vi "Init and Rotate array Graf3.vi"(5 "Reset":bool, 7 "Stop read":bool, 9 "Array size":i32=30, 10 "PV":dbl[](array[numeric]), 11 "XY Graf in":cluster{"time stamp":timestamp[], "PV":dbl[]}[](array[cluster])) -> (3 "XY Graf out":cluster{"time stamp":timestamp[], "PV":dbl[]}[](array[cluster]))   [LabVIEW 2019]
panel:
  out "XY Graf out 2":cluster{"time stamp":timestamp[], "PV":dbl[]}[](array[cluster])
  in  "XY Graf in 2":cluster{"time stamp":timestamp[], "PV":dbl[]}[](array[cluster])
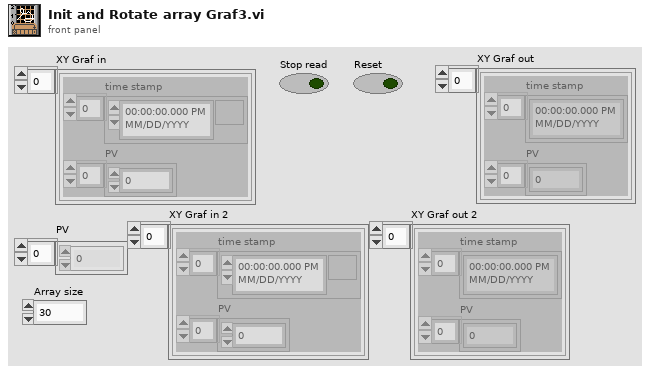
[diagram p1: front panel]
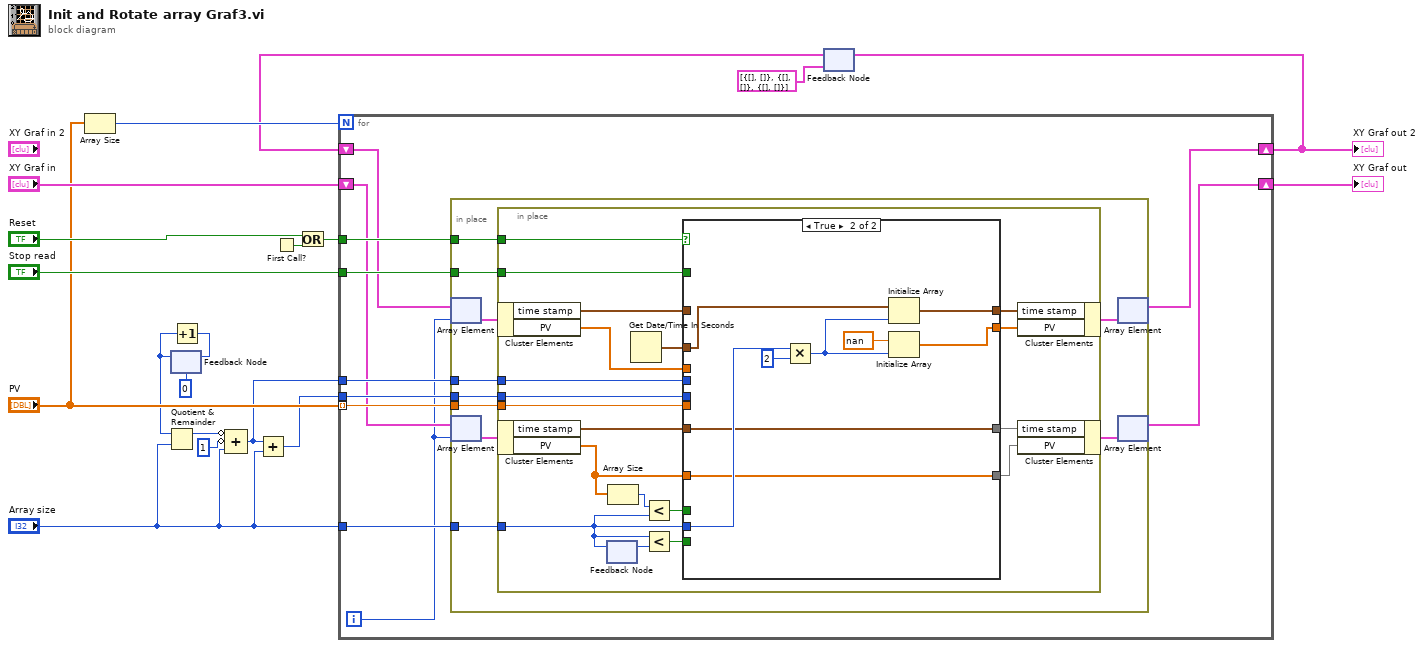
[diagram p0: block diagram]
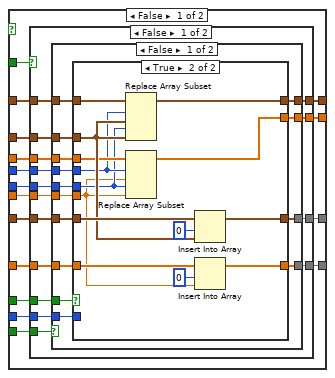
[diagram p2: hidden frame]
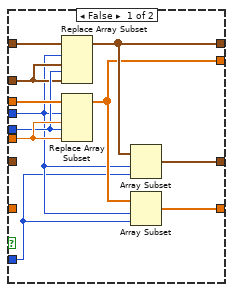
[diagram p3: hidden frame]
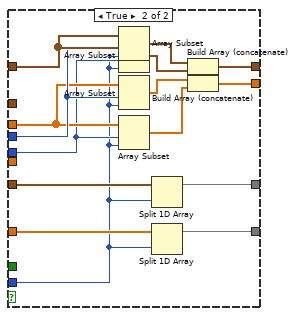
[diagram p4: hidden frame]
diagram:
  n1 = Array Size(array="PV") -> (size(s)=w15:i32)
  n2 = feedback #1(0 ("t")) -> (w11:i32)
  n3 = Quotient & Remainder(x=w11, y="Array size") -> (x-y*floor(x/y)=w10:i32)  [unwired: 1 out]
  n4 = Increment(x=w11) -> (x+1=w12:i32)
  n5 = feedback-in #1(w12) -> ()
  n6 = Compound Arithmetic op=ADD(invert w10, invert 1 ("value"), "Array size") -> (w7:i32)
  n7 = Add(x=w7, y="Array size") -> (x+y=w6:i32)
  n8 = First Call?() -> (First Call?: T/F=w4:bool)
  n9 = Or(x="Reset", y=w4) -> (x .or. y?=w5:bool)
  n10 = feedback #2(cluster{"time stamp":timestamp[], "PV":dbl[]}[] [{"time stamp"=[], "PV"=[]}, {"time stamp"=[], "PV"=[]}, {"time stamp"=[], "PV"=[]}] ("XY Graf out")) -> (w2:cluster{"time stamp":timestamp[], "PV":dbl[]}[])
  n11 = for {
    N: w15 -> [_]
    tunnel: "Stop read" -> [w30]
    tunnel: w5 -> [w29]
    tunnel: "PV" -> [w28] mode=indexing
    tunnel: "Array size" -> [w27]
    shift-right: [w20] -> w17
    shift-left: "XY Graf in" -> [w24]
    shift-right: [w21] -> w3
    shift-left: w2 -> [w23]
    tunnel: w7 -> [w26]
    tunnel: w6 -> [w25]
    i -> [w22]
    n12 = in-place {
      in-place-border: w30 -> [w40]
      in-place-border: w29 -> [w39]
      in-place-border: w28 -> [w38]
      in-place-border: w27 -> [w37]
      in-place-border: w26 -> [w36]
      in-place-border: w25 -> [w35]
      n13 = in-place-array #3(w23, w22) -> (w32:cluster{"time stamp":timestamp[], "PV":dbl[]})
      n14 = in-place-array #4(w24, w22) -> (w33:cluster{"time stamp":timestamp[], "PV":dbl[]})
      n15 = in-place {
        in-place-border: w40 -> [w59]
        in-place-border: w39 -> [w54]
        in-place-border: w38 -> [w57]
        in-place-border: w37 -> [w50]
        in-place-border: w36 -> [w44]
        in-place-border: w35 -> [w43]
        n16 = in-place-cluster #5(w32) -> ("time stamp"=w46:timestamp[], "PV"=w42:dbl[])
        n17 = in-place-cluster #6(w33) -> ("time stamp"=w55:timestamp[], "PV"=w49:dbl[])
        n18 = feedback #7() -> (w53:i32)  [unwired: 1 in]
        n19 = feedback-in #7(w50) -> ()
        n20 = Array Size(array=w49) -> (size(s)=w58:i32)
        n21 = Get Date/Time In Seconds() -> (seconds since 1Jan1904=w56:timestamp)
        n22 = Less?(x=w58, y=w50) -> (x < y?=w48:bool)
        n23 = Less?(x=w50, y=w53) -> (x < y?=w52:bool)
        n24 = case shown="True" w54 {
          tunnel: w59 -> [w67 _]
          tunnel: w57 -> [w75 _]
          tunnel: w56 -> [w74 w157]
          tunnel: [w73 w150] -> w51
          tunnel: w55 -> [w72 w150]
          tunnel: w49 -> [w71 w149]
          tunnel: [w70 w149] -> w47
          tunnel: w52 -> [w66 _]
          tunnel: w50 -> [w69 w156]
          tunnel: w48 -> [w68 _]
          tunnel: w46 -> [w65 _]
          tunnel: [w64 w152] -> w45
          tunnel: w44 -> [w63 _]
          tunnel: w43 -> [w62 _]
          tunnel: w42 -> [w61 _]
          tunnel: [w60 w153] -> w41
          frame False {
            n25 = case shown="False" w67 {
              tunnel: w66 -> [w84 _]
              tunnel: w75 -> [w90 _]
              tunnel: w74 -> [w89 _]
              tunnel: [w88 w148] -> w73
              tunnel: w72 -> [w87 w148]
              tunnel: w71 -> [w86 w147]
              tunnel: [w85 w147] -> w70
              tunnel: w69 -> [w82 _]
              tunnel: w68 -> [w83 _]
              tunnel: w65 -> [w81 w146]
              tunnel: [w80 w146] -> w64
              tunnel: w63 -> [w79 _]
              tunnel: w62 -> [w78 _]
              tunnel: w61 -> [w77 w145]
              tunnel: [w76 w145] -> w60
              frame False {
                n26 = case shown="False" w84 {
                  tunnel: w90 -> [w104 _]
                  tunnel: w89 -> [w103 _]
                  tunnel: w87 -> [w102 w143]
                  tunnel: w86 -> [w101 w144]
                  tunnel: [w100 w141] -> w85
                  tunnel: [w99 w142] -> w88
                  tunnel: w83 -> [w98 _]
                  tunnel: w82 -> [w91 w136]
                  tunnel: w81 -> [w97 w140]
                  tunnel: [w96 w133] -> w80
                  tunnel: w79 -> [w95 w139]
                  tunnel: w78 -> [w94 w137]
                  tunnel: w77 -> [w93 w138]
                  tunnel: [w92 w130] -> w76
                  frame False {
                    n27 = case shown="True" w98 {
                      tunnel: w102 -> [_ w127]
                      tunnel: w103 -> [w111 w122]
                      tunnel: w101 -> [_ w126]
                      tunnel: w104 -> [w113 w116]
                      tunnel: [w109 w125] -> w99
                      tunnel: [w107 w124] -> w100
                      tunnel: w97 -> [w115 w123]
                      tunnel: [w110 w121] -> w96
                      tunnel: w95 -> [w106 w119]
                      tunnel: w94 -> [w112 w118]
                      tunnel: w93 -> [w114 w120]
                      tunnel: [w108 w117] -> w92
                      tunnel: w91 -> [w105 _]
                      frame False {
                        n28 = Replace Array Subset(array=w115, new element #1=w111, index #1=w106, new element #2=w111, index #2=w112) -> (w110:timestamp[])
                        n29 = Replace Array Subset(array=w114, new element #1=w113, index #1=w106, new element #2=w113, index #2=w112) -> (w108:dbl[])
                        n30 = Array Subset(array=w110, index=w106, length=w105) -> (w109:timestamp[])
                        n31 = Array Subset(array=w108, index=w106, length=w105) -> (w107:dbl[])
                      }
                      frame True {
                        n32 = Replace Array Subset(array=w123, new element #1=w122, index #1=w119, new element #2=w122, index #2=w118) -> (w121:timestamp[])
                        n33 = Replace Array Subset(array=w120, new element #1=w116, index #1=w119, new element #2=w116, index #2=w118) -> (w117:dbl[])
                        n34 = Insert Into Array(array=w127, index=0, new element=w122) -> (w125:timestamp[])
                        n35 = Insert Into Array(array=w126, index=0, new element=w116) -> (w124:dbl[])
                      }
                    }
                  }
                  frame True {
                    n36 = Array Subset(array=w140, index=w139, length=w136) -> (w135:timestamp[])
                    n37 = Array Subset(array=w140, index=w137, length=w136) -> (w134:timestamp[])
                    n38 = Array Subset(array=w138, index=w139, length=w136) -> (w132:dbl[])
                    n39 = Array Subset(array=w138, index=w137, length=w136) -> (w131:dbl[])
                    n40 = Split 1D Array(array=w143, index=w136) -> (first subarray=w142:timestamp[])  [unwired: 1 out]
                    n41 = Split 1D Array(array=w144, index=w136) -> (first subarray=w141:dbl[])  [unwired: 1 out]
                    n42 = Build Array (concatenate)(w135, w134) -> (w133:timestamp[])
                    n43 = Build Array (concatenate)(w132, w131) -> (w130:dbl[])
                  }
                }
              }
              frame True {
              }
            }
          }
          frame True {
            n44 = Multiply(x=w156, y=2) -> (x*y=w151:i32)
            n45 = Initialize Array(w157, w151) -> (w152:timestamp[])
            n46 = Initialize Array(nan ("PV"), w151) -> (w153:dbl[])
          }
        }
        n47 = in-place-cluster #5("time stamp"=w45, "PV"=w41) -> (w31:cluster{"time stamp":timestamp[], "PV":dbl[]})
        n48 = in-place-cluster #6("time stamp"=w51, "PV"=w47) -> (w34:cluster{"time stamp":timestamp[], "PV":dbl[]})
      }
      n49 = in-place-array #3(w31) -> (w21:cluster{"time stamp":timestamp[], "PV":dbl[]}[])  [unwired: 1 out]
      n50 = in-place-array #4(w34) -> (w20:cluster{"time stamp":timestamp[], "PV":dbl[]}[])  [unwired: 1 out]
    }
  }
  "XY Graf out" <- w17
  "XY Graf out 2" <- w3
  n51 = feedback-in #2(w3) -> ()
